vi "vi.CreateDBLArray.vi"() -> ()   [LabVIEW 2014, in "GLue.lvlib" / "class.GLue.lvclass"]
uses:
  class.GLue.lvclass
panel:
  out "DBLArray":dbl[][](array[numeric])
  in  "Columns":i32
  in  "Rows":i32
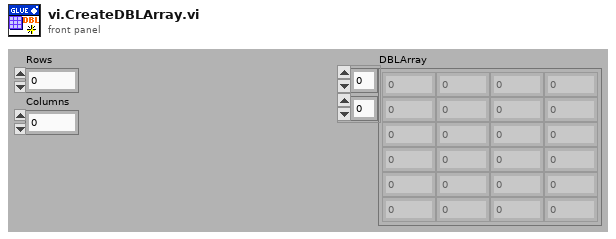
[diagram p1: front panel]
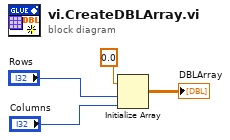
[diagram p0: block diagram]
diagram:
  n1 = Initialize Array(0.0 ("element"), "Rows", "Columns") -> (→"DBLArray":dbl[][])
